vi "Close Spectrum Reader.vi"(8 "error in (no error)":errorcluster, 11 "endpoint in":refnum<k21>) -> (0 "error out":errorcluster)   [LabVIEW 2017]
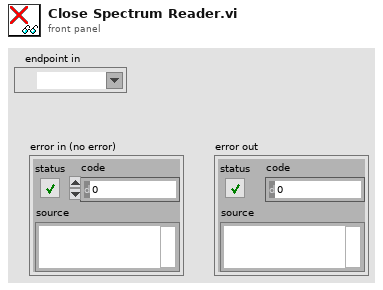
[diagram p1: front panel]
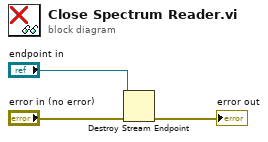
[diagram p0: block diagram]
diagram:
  n1 = Destroy Stream Endpoint(8:"error in (no error)", 11:"endpoint in") -> (0:→"error out":errorcluster)
